vi "DSF.Engine.Interface.Read.Command.vi"(8 "error in (no error)":errorcluster, 9 "timeout in ms (0)":i32, 11 "Interface in":refnum<class "DSF.Engine.Interface.lvclass">) -> (0 "error out":errorcluster, 1 "timed out?":bool, 2 "command":T1, 3 "Interface out":refnum<class "DSF.Engine.Interface.lvclass">, 4 "# elements":u32)   [LabVIEW 2017, in "Data Sharing Framework Engine.lvlib" / "DSF.Engine.Interface.lvclass"]
uses:
  DSF.Engine.Interface.lvclass
  DSF.Engine.Interface.RT FIFO.Data.16B.ctl
  DSF.Engine.Interface.RT FIFO.Payload.16B.ctl
  DSF.Engine.Interface.lvclass/DSF.Engine.Interface.ctl
  Debug/DSF.Engine.Debug Flags.FIFO.lvclass/DSF.Engine.Debug Flags.FIFO.ctl
  Debug/DSF.Engine.Debug Flags.FIFO.Get Infinite Timeouts.vi
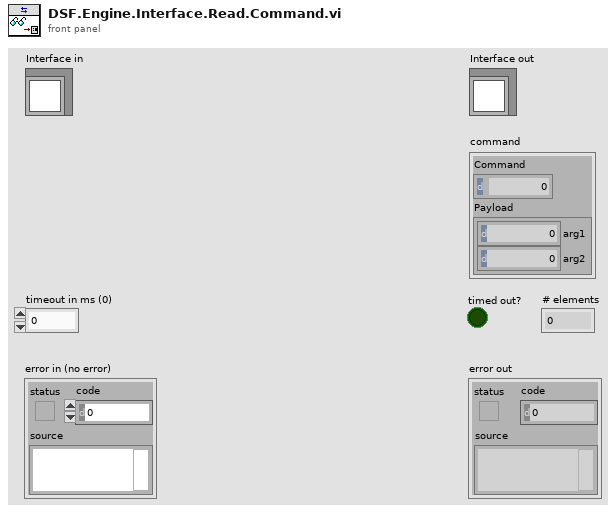
[diagram p1: front panel]
types:
  T1 = typedef "Data Sharing Framework Engine.lvlib/DSF.Engine.Interface.lvclass/DSF.Engine.Interface.RT FIFO.Data.16B.ctl" = cluster{"Command":u8, "Payload":T2}
  T2 = typedef "Data Sharing Framework Engine.lvlib/DSF.Engine.Interface.lvclass/DSF.Engine.Interface.RT FIFO.Payload.16B.ctl" = cluster{"arg1":u64, "arg2":u64}
  T3 = typedef "Data Sharing Framework Engine.lvlib/DSF.Engine.Interface.lvclass/DSF.Engine.Interface.RT FIFO.Ref.16B.ctl" = refnum<k33>
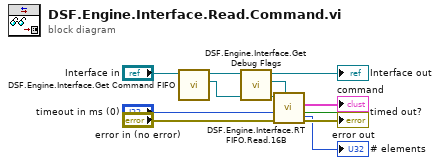
[diagram p0: block diagram]
diagram:
  n1 = call "DSF.Engine.Interface.Get Command FIFO.vi"("Interface in"="Interface in") -> ("Command FIFO"=w11:T3, "Interface out"=w7:refnum<class "DSF.Engine.Interface.lvclass">)  [unwired: 9 in]
  n2 = call "DSF.Engine.Interface.Get Debug Flags.vi"("Interface in"=w7) -> ("FIFO Debug Flags"=w6:refnum<class "DSF.Engine.Debug Flags.FIFO.lvclass">, "Interface out"=→"Interface out":refnum<class "DSF.Engine.Interface.lvclass">)  [unwired: 9 in]
  n3 = call "DSF.Engine.Interface.RT FIFO.Read.16B.vi"("FIFO Debug Flags"=w6, "error in (no error)"="error in (no error)", "timeout in ms (0)"="timeout in ms (0)", "RT FIFO in"=w11) -> ("error out"=→"error out":errorcluster, "empty?"=→"timed out?":bool, "element out"=→"command":T1, "# elements"=→"# elements":u32)  [unwired: 3 in, 1 out]
